vi "FTW-CodeGen-XNodeReply.vi"(0 "XNode Reply Type":T1, 11 "error in":errorcluster) -> (4 "Reply":string[](array[string]))   [LabVIEW 2014]
uses:
  FTW-CodeGen-XNodeReplyType.ctl
panel:
  # "Inputs"
  # "Outputs"
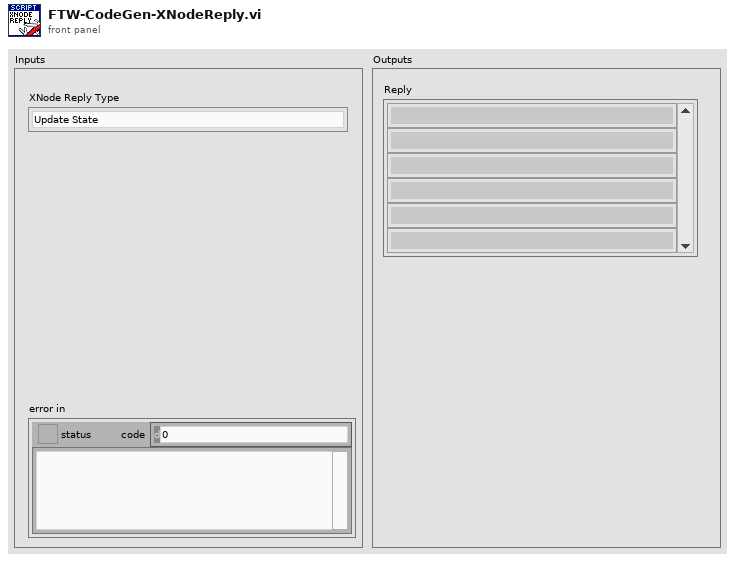
[diagram p1: front panel]
types:
  T1 = typedef "FTW-CodeGen-XNodeReplyType.ctl" = enum16{"Update State", "AdaptToInputs", "CosmeticUpdate", "No Reply"}
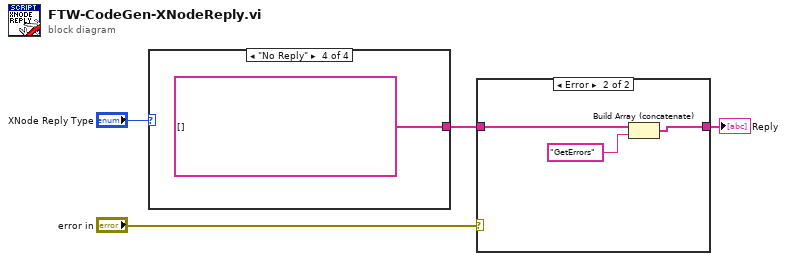
[diagram p0: block diagram]
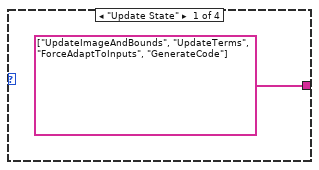
[diagram p3: hidden frame]
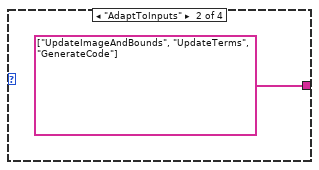
[diagram p4: hidden frame]
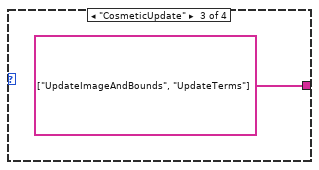
[diagram p5: hidden frame]
diagram:
  n1 = case shown="\"No Reply\"" "XNode Reply Type" {
    tunnel: [string[] ["UpdateImageAndBounds", "UpdateTerms", "ForceAdaptToInputs", "GenerateCode"] ("Reply") string[] ["UpdateImageAndBounds", "UpdateTerms", "GenerateCode"] ("Reply") string[] ["UpdateImageAndBounds", "UpdateTerms"] ("Reply") string[] [] ("Reply")] -> w1
    frame "Update State" {
    }
    frame "AdaptToInputs" {
    }
    frame "CosmeticUpdate" {
    }
    frame "No Reply" {
    }
  }
  n2 = case shown="Error" "error in" {
    tunnel: [w9 w11] -> w2
    tunnel: w1 -> [w9 w12]
    frame No Error {
    }
    frame Error {
      n3 = Build Array (concatenate)(w12, "GetErrors") -> (w11:string[])
    }
  }
  "Reply" <- w2
